vi "Main.vi"() -> ()   [LabVIEW 2016]
uses:
  <vilib>/LabVIEW Interface for Arduino/Type Defs/Board Type.ctl
  <vilib>/Utility/file.llb/Write Delimited Spreadsheet (string).vi
  <vilib>/LabVIEW Interface for Arduino/LabVIEW Interface for Arduino.lvlib
panel:
  out "error out 2":errorcluster
  out "Raw Data":dbl[](graph)
  out "Vout to save":dbl[](graph)
  in  "Gain":dbl=99.0 format="%#_13g"
  out "Data":dbl[](array[numeric])
  in  "Analog Input Pin":u8
  in  "Acquition Speed":u32
  in  "Filename":path=path "D:/do an nang cao/data.xlsx"
  out "error out":errorcluster
  in  "VISA resource":refnum<visa-resource-name>
  in  "stop":bool
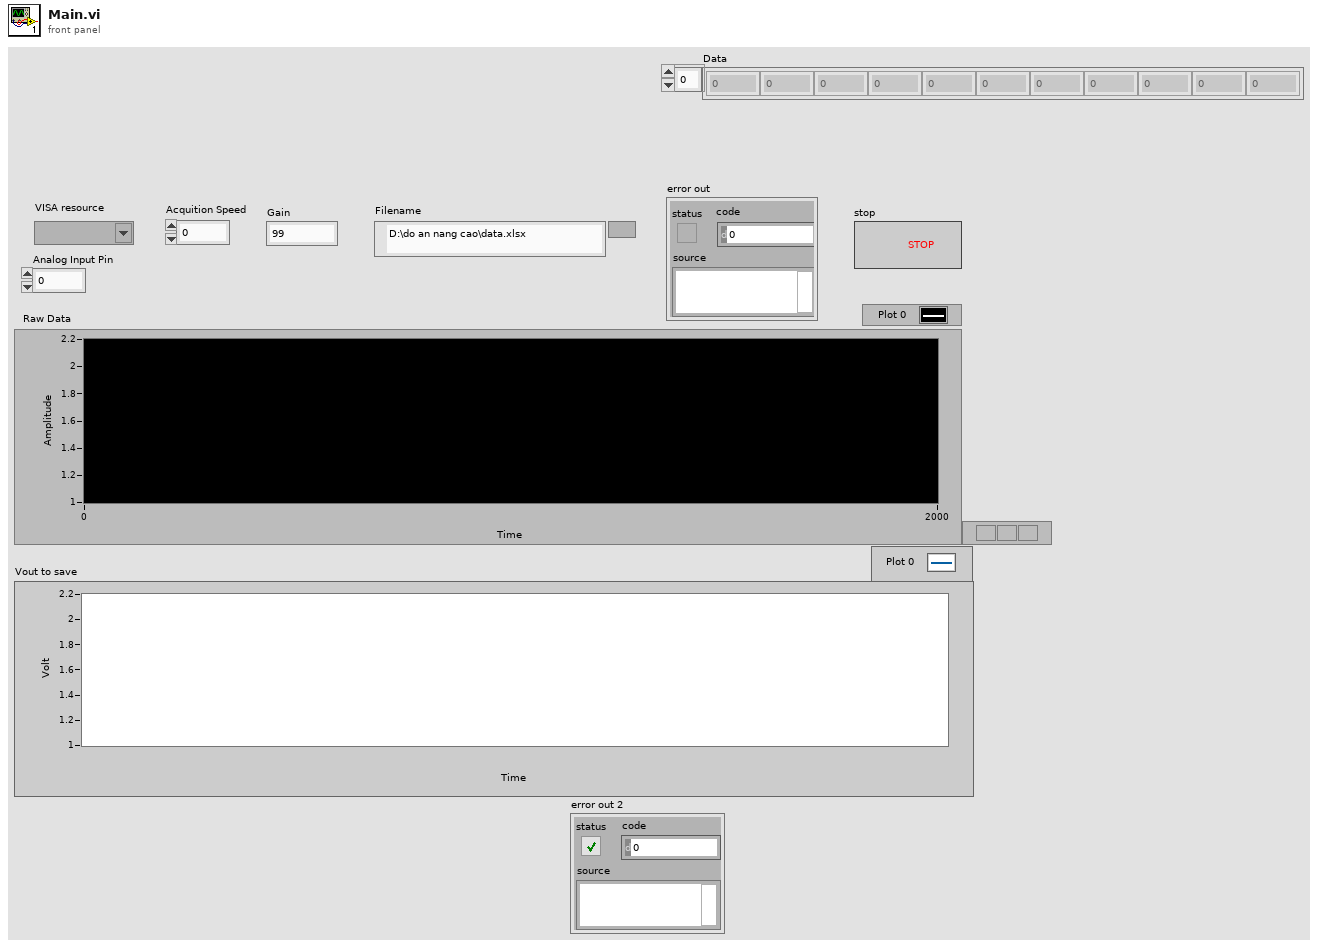
[diagram p1: front panel]
types:
  T1 = typedef "LabVIEW Interface for Arduino.lvlib/Board Type.ctl" = enum16{"Uno", "Dimuelanove w/Atmega 328", "Mega 2560"}
  T2 = typedef "LabVIEW Interface for Arduino.lvlib/Arduino Resource.ctl" = cluster{"VISA resource":refnum<visa-resource-name>, "Board Type":T1, "Connection Type":enum8{"USB / Serial"}, "Bytes Per Packet (15)":u8}
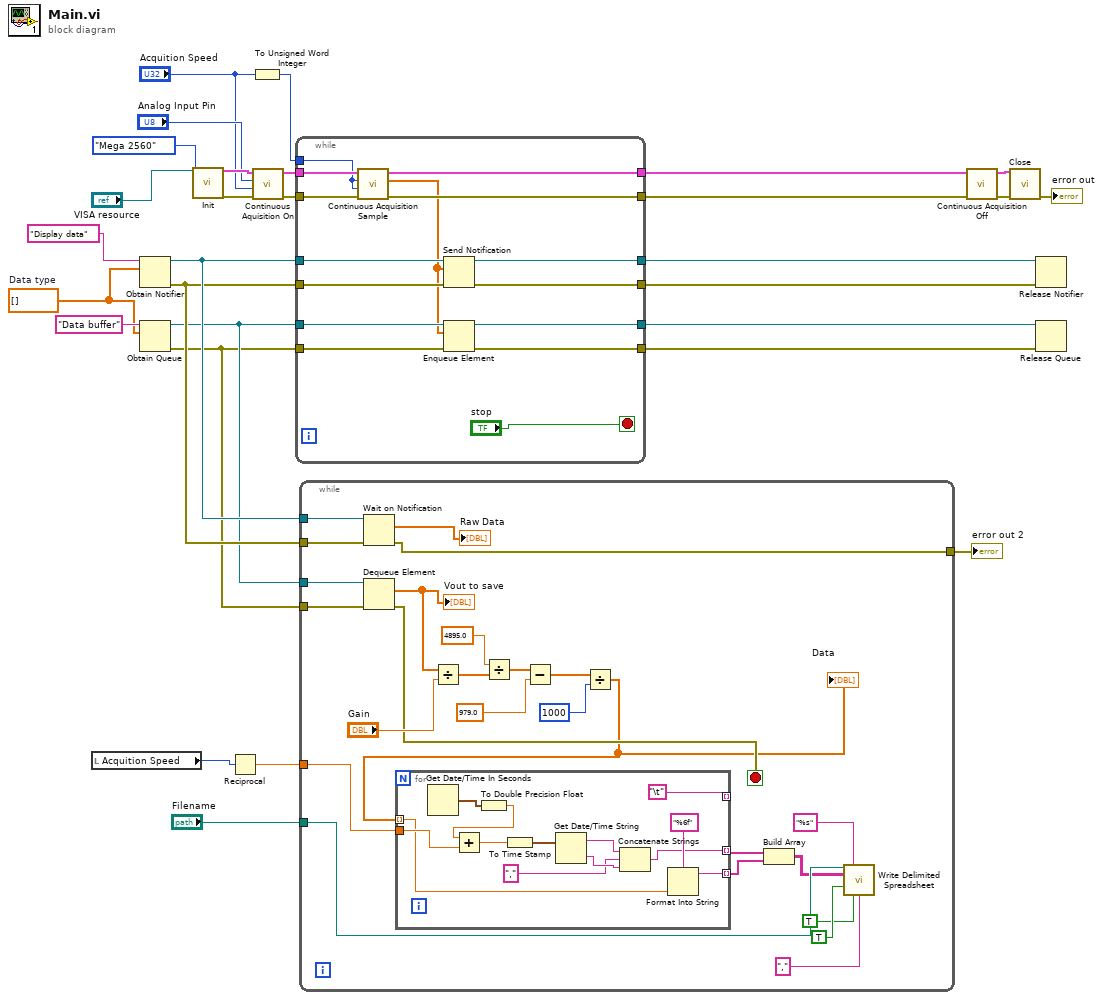
[diagram p0: block diagram]
diagram:
  w13 = dbl[] []  # Data type
  n1 = local read "Acquition Speed"() -> (w2:u32)
  n2 = Obtain Notifier(name (unnamed)="Display data", notification data type=w13) -> (notifier out=w10:refnum<notifier>, error out=w9:errorcluster)  [unwired: 2 in, 1 out]
  n3 = Obtain Queue(name (unnamed)="Data buffer", element data type=w13) -> (queue out=w8:refnum<queue>, error out=w7:errorcluster)  [unwired: 3 in, 1 out]
  n4 = call <vilib>:"Init.vi"("VISA resource"="VISA resource", "Board Type (Uno)"=Board_Type."Mega 2560") -> ("Arduino Resource"=w29:T2, "error out"=w25:errorcluster)  [unwired: 16 in]
  n5 = Reciprocal(x=w2) -> (1/x=w1:dbl)
  n6 = To Unsigned Word Integer(number="Acquition Speed") -> (unsigned 16bit integer=w19:u16)
  n7 = call <vilib>:"Continuous Aquisition On.vi"("error in"=w25, "Acquition Speed"="Acquition Speed", "Analog Input Pin"="Analog Input Pin", "Arduino Resource"=w29) -> ("error out"=w24:errorcluster, "Arduino Resource"=w28:T2)  [unwired: 6 in]
  n8 = while {
    tunnel: w28 -> [w44]
    tunnel: [w43] -> w27
    tunnel: w24 -> [w42]
    tunnel: [w41] -> w23
    tunnel: w19 -> [w39]
    tunnel: w10 -> [w38]
    tunnel: w9 -> [w37]
    tunnel: [w36] -> w15
    tunnel: [w35] -> w5
    tunnel: w8 -> [w34]
    tunnel: [w33] -> w12
    tunnel: [w32] -> w11
    tunnel: w7 -> [w31]
    stop <- "stop" stop-if-true
    n9 = call <vilib>:"Continuous Acquisition Sample.vi"("Arduino Resource"=w44, "Samples to Read"=w39, "Sample Rate (HZ)"=w39, "error in (no error)"=w42) -> ("Arduino Resource"=w43:T2, "Data"=w30:dbl[], "error out"=w41:errorcluster)  [unwired: 4 in]
    n10 = Send Notification(notification=w30, notifier=w38, error in (no error)=w37) -> (notifier out=w36:refnum<notifier>, error out=w35:errorcluster)
    n11 = Enqueue Element(queue=w34, element=w30, error in (no error)=w31) -> (queue out=w33:refnum<queue>, error out=w32:errorcluster)  [unwired: 1 in, 1 out]
  }
  n12 = while {
    tunnel: w10 -> [w69]
    tunnel: w9 -> [w68]
    tunnel: w8 -> [w66]
    tunnel: w7 -> [w65]
    tunnel: [w64] -> w4
    tunnel: "Filename" -> [w52]
    tunnel: w1 -> [w54]
    stop <- w55 stop-if-true
    n13 = Wait on Notification(notifier=w69, error in (no error)=w68) -> (notification=→"Raw Data":dbl[], error out=w64:errorcluster)  [unwired: 2 in, 2 out]
    n14 = Dequeue Element(queue=w66, error in (no error)=w65) -> (element=w56:dbl[], error out=w55:errorcluster)  [unwired: 1 in, 2 out]
    "Vout to save" <- w56
    n15 = Divide(x=w56, y="Gain") -> (x/y=w58:dbl[])
    n16 = Divide(x=4895.0, y=w58) -> (x/y=w60:dbl[])
    n17 = Subtract(x=w60, y=979.0 ("x")) -> (x-y=w62:dbl[])
    n18 = Divide(x=w62, y=1000) -> (x/y=w48:dbl[])
    "Data" <- w48
    n19 = for {
      tunnel: w48 -> [w79] mode=indexing
      tunnel: w54 -> [w80]
      tunnel: [w73] -> w45 mode=indexing
      tunnel: [w72] -> w49 mode=indexing
      tunnel: ["\t"] -> _ mode=indexing
      n20 = Get Date/Time In Seconds() -> (seconds since 1Jan1904=w82:timestamp)
      n21 = To Double Precision Float(number=w82) -> (double precision float=w81:dbl)
      n22 = Add(x=w81, y=w80) -> (x+y=w77:dbl)
      n23 = To Time Stamp(1:w77) -> (0:w76:timestamp)
      n24 = Get Date/Time String(seconds (now)=w76) -> (date string=w75:string, time string=w74:string)  [unwired: 2 in]
      n25 = Concatenate Strings(w75, ",", w74) -> (w72:string)
      n26 = Format Into String(format string="%6f", w79) -> (resulting string=w73:string)  [unwired: 2 in, 1 out]
    }
    n27 = Build Array(w49, w45) -> (w47:string[][])
    n28 = call-poly <vilib>:"Write Delimited Spreadsheet.vi"("file path (dialog if empty)"=w52, "format (%s)"="%s" ("format (%.3f)"), "2D data"=w47, "append to file? (new file:F)"=TRUE, "transpose? (no:F)"=TRUE, "delimiter (\\t)"="," ("delimiter (\\t)")) -> ()  [unwired: 8 in, 2 out]
  }
  "error out 2" <- w4
  n29 = call <vilib>:"Continuous Acquisition Off.vi"("error in"=w23, "Arduino Resource"=w27) -> ("error out"=w22:errorcluster, "Arduino Resource"=w26:T2)  [unwired: 8 in]
  n30 = call <vilib>:"Close.vi"("Arduino Resource"=w26, "error in"=w22) -> ("error out"=→"error out":errorcluster)  [unwired: 13 in]
  n31 = Release Notifier(notifier=w15, error in (no error)=w5) -> ()  [unwired: 1 in, 3 out]
  n32 = Release Queue(queue=w12, error in (no error)=w11) -> ()  [unwired: 1 in, 3 out]
